vi "Set Channel.vi"(8 "error in (no error)":errorcluster, 10 "Channel Parameters":T1={"Channel"=enum."Channel 2", "Gain"=enum."10x", "Input Config"=enum."Differential", "Shunt Resistor"=enum."50 Ohms", "Coupling"=enum."DC", "Bandwidth Filter"=enum."ON"}, 11 "VISA Refnum in":refnum<visa-resource-name>="COM1") -> (0 "error out":errorcluster, 3 "VISA Refnum out":refnum<visa-resource-name>)   [LabVIEW 2019, in "KH7008.lvlib"]
uses:
  KH7008.lvlib
  Inst.Krohn-Hite-7008/Typedefs/SetAll-Cluster.ctl
  Inst.Krohn-Hite-7008/Typedefs/Channel-Enum.ctl
  Inst.Krohn-Hite-7008/Typedefs/Gain-Enum.ctl
  Inst.Krohn-Hite-7008/Typedefs/Input Configuration-Enum.ctl
  Inst.Krohn-Hite-7008/Typedefs/Shunt-Enum.ctl
  Inst.Krohn-Hite-7008/Typedefs/Coupling-Enum.ctl
  Inst.Krohn-Hite-7008/Typedefs/Filter-Enum.ctl
  Inst.Krohn-Hite-7008/Inst.Krohn-Hite-7008.lvclass
panel:
  out "Response":string
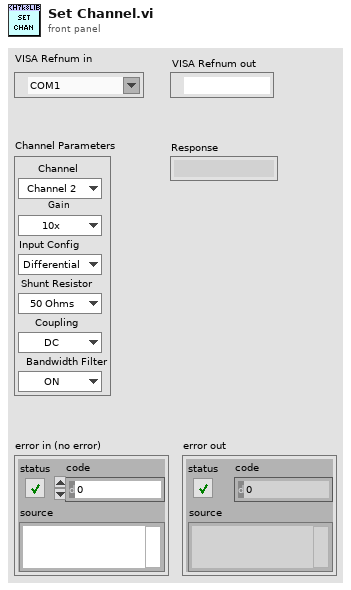
[diagram p1: front panel]
types:
  T1 = typedef "Inst.Krohn-Hite-7008.lvclass/SetAll-Cluster.ctl" = cluster{"Channel":T2, "Gain":T3, "Input Config":T4, "Shunt Resistor":T5, "Coupling":T6, "Bandwidth Filter":T7}
  T2 = typedef "Inst.Krohn-Hite-7008.lvclass/Channel-Enum.ctl" = enum16{"Channel 1", "Channel 2", "Channel 3", "Channel 4", "Channel 5", "Channel 6", "Channel 7", "Channel 8"}
  T3 = typedef "Inst.Krohn-Hite-7008.lvclass/Gain-Enum.ctl" = enum16{"1x", "10x", "100x", "1000x"}
  T4 = typedef "Inst.Krohn-Hite-7008.lvclass/Input Configuration-Enum.ctl" = enum16{"Ground", "SE+ (-gnd)", "SE- (+gnd)", "Differential"}
  T5 = typedef "Inst.Krohn-Hite-7008.lvclass/Shunt-Enum.ctl" = enum16{"Open", "50 Ohms", "500 Ohms", "5k Ohms", "50k Ohms", "10M Ohm"}
  T6 = typedef "Inst.Krohn-Hite-7008.lvclass/Coupling-Enum.ctl" = enum16{"AC", "DC"}
  T7 = typedef "Inst.Krohn-Hite-7008.lvclass/Filter-Enum.ctl" = enum16{"OFF", "ON"}
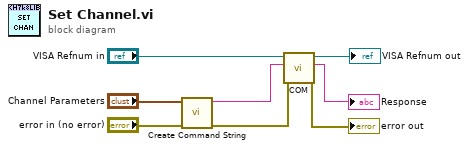
[diagram p0: block diagram]
diagram:
  n1 = call "Create Command String.vi"("error in (no error)"="error in (no error)", "Channel Params"="Channel Parameters") -> ("error out"=w4:errorcluster, "Command string"=w1:string)  [unwired: 8 in]
  n2 = call "COM.vi"("error in (no error)"=w4, "Command"=w1, "VISA Refnum in"="VISA Refnum in") -> ("error out"=→"error out":errorcluster, "Response"=→"Response":string, "VISA Refnum out"=→"VISA Refnum out":refnum<visa-resource-name>)  [unwired: 6 in]
